vi "CreateABLEDataStructures.vi"(8 "Error In":errorcluster) -> (0 "Error Out":errorcluster, 3 "ABLE Data Structures":T1)   [LabVIEW 2012]
uses:
  ABLEDataStructures.ctl
  HardwareDisplayData.ctl
  BPM.ctl
  ExperimentHardwareData.ctl
  ExperimentData.ctl
  AlarmData.ctl
  AlarmDatum.ctl
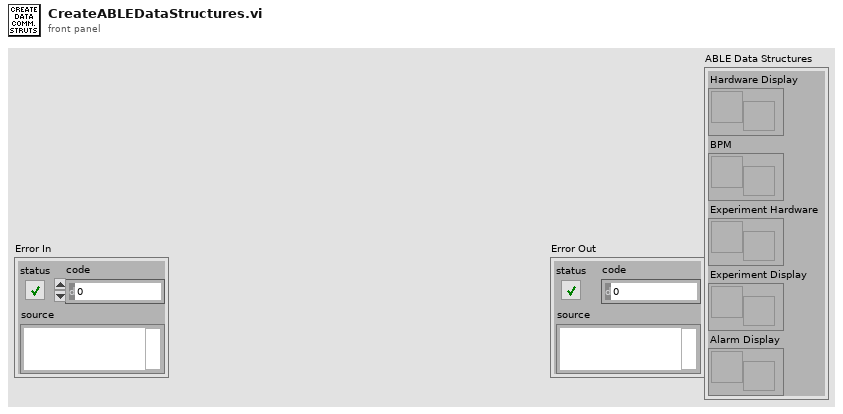
[diagram p1: front panel]
types:
  T1 = typedef "ABLEDataStructures.ctl" = cluster{"Hardware Display":refnum<notifier>, "BPM":refnum<notifier>, "Experiment Hardware":refnum<notifier>, "Experiment Display":refnum<notifier>, "Alarm Display":refnum<notifier>}
  T2 = typedef "AlarmData.ctl" = cluster{"Temperature":T3[]}
  T3 = typedef "AlarmDatum.ctl" = cluster{"Actual":dbl, "Activated?":bool}
  T4 = typedef "ExperimentData.ctl" = cluster{"Flux (ions/s * cm^2)":dbl, "Average Flux (ions/s * cm^2)":dbl, "DPA Rate":dbl, "Average DPA Rate":dbl, "Total Ion Energy (MeV)":dbl, "Total Charge (C)":dbl, "Dose (DPA)":dbl, "Fluence (ions/cm^2)":dbl, "Percent Complete (%)":dbl, "Duration (sec)":dbl}
  T5 = typedef "ExperimentHardwareData.ctl" = cluster{"Beam Current (A)":dbl, "Terminal Voltage (MeV)":dbl}
  T6 = typedef "HardwareDisplayData.ctl" = cluster{"Temperatures (C)":dbl[], "Terminal Voltage (MeV)":dbl, "Currents (A)":dbl[]}
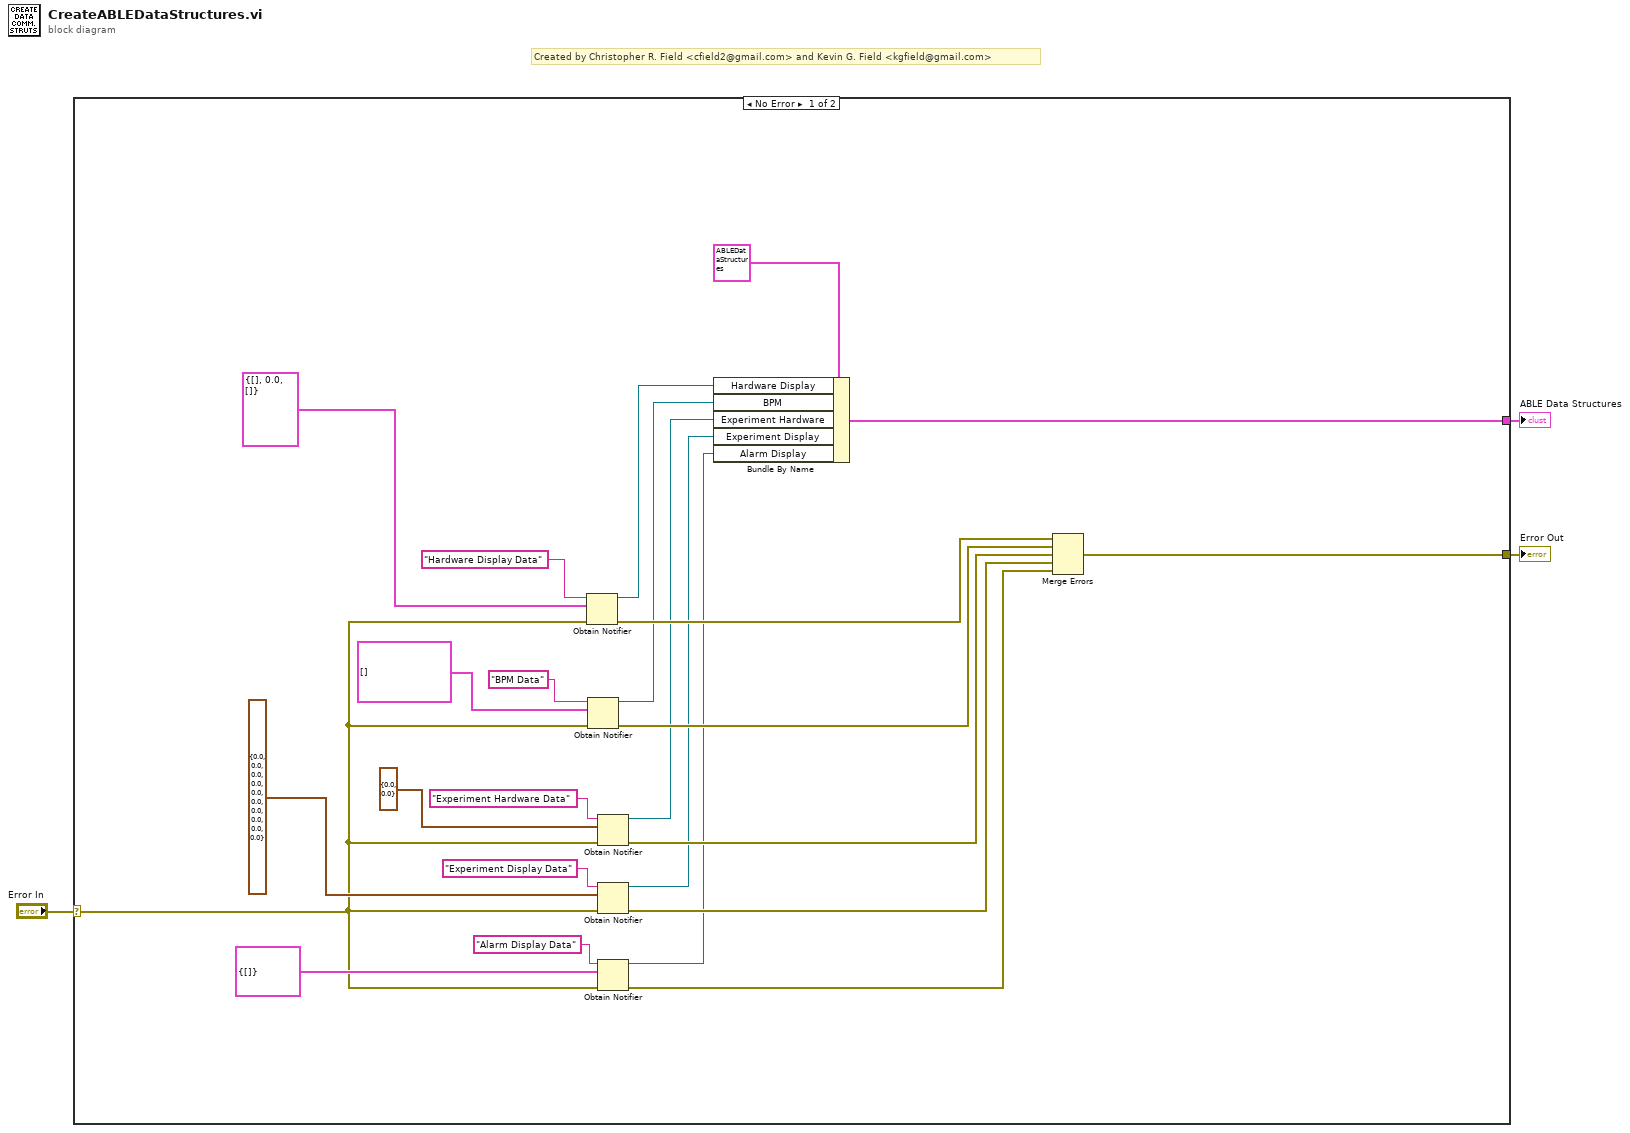
[diagram p0: block diagram]
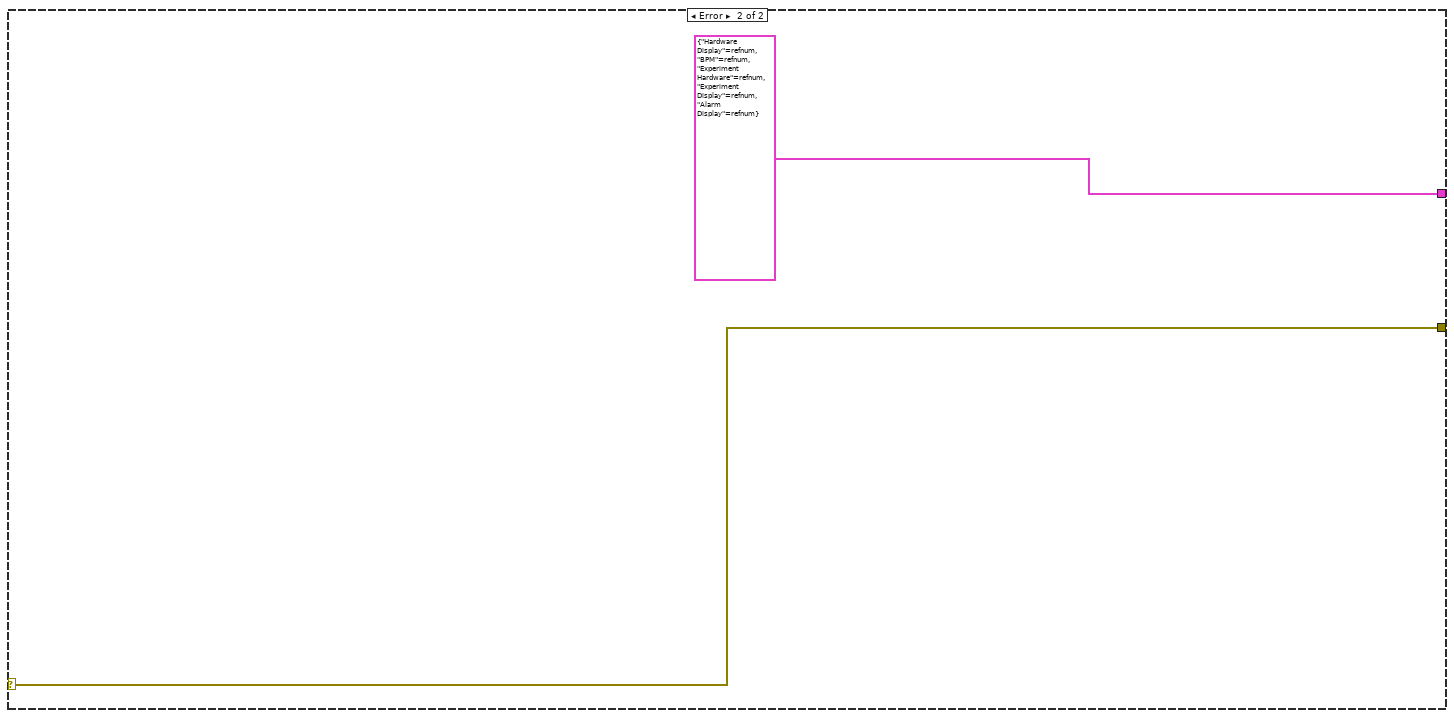
[diagram p2: hidden frame]
diagram:
  # "Created by Christopher R. Field <cfield2@gmail.com> and Kevin G. Field <kgfield@gmail.com>"
  n1 = case shown="No Error" "Error In" {
    selector: "Error In" -> [w6 w29]
    tunnel: [w26 w29] -> w2
    tunnel: [w24 T1 {"Hardware Display"=refnum, "BPM"=refnum, "Experiment Hardware"=refnum, "Experiment Display"=refnum, "Alarm Display"=refnum} ("Data Communication Structures")] -> w1
    frame No Error {
      n2 = Obtain Notifier(name (unnamed)="Hardware Display Data", notification data type=T6 {"Temperatures (C)"=[], "Terminal Voltage (MeV)"=0.0, "Currents (A)"=[]} ("Display Data"), error in (no error)=w6) -> (notifier out=w17:refnum<notifier>, error out=w23:errorcluster)  [unwired: 1 in, 1 out]
      n3 = Obtain Notifier(name (unnamed)="BPM Data", notification data type=cluster{dbl[], "Beam Profile":dbl[]}[] [] ("BPM"), error in (no error)=w6) -> (notifier out=w20:refnum<notifier>, error out=w21:errorcluster)  [unwired: 1 in, 1 out]
      n4 = Obtain Notifier(name (unnamed)="Experiment Hardware Data", notification data type=T5 {"Beam Current (A)"=0.0, "Terminal Voltage (MeV)"=0.0} ("Experiment Hardware Data"), error in (no error)=w6) -> (notifier out=w11:refnum<notifier>, error out=w14:errorcluster)  [unwired: 1 in, 1 out]
      n5 = Obtain Notifier(name (unnamed)="Experiment Display Data", notification data type=T4 {"Flux (ions/s * cm^2)"=0.0, "Average Flux (ions/s * cm^2)"=0.0, "DPA Rate"=0.0, "Average DPA Rate"=0.0, "Total Ion Energy (MeV)"=0.0, "Total Charge (C)"=0.0, "Dose (DPA)"=0.0, "Fluence (ions/cm^2)"=0.0, "Percent Complete (%)"=0.0, "Duration (sec)"=0.0} ("Experiment Data"), error in (no error)=w6) -> (notifier out=w9:refnum<notifier>, error out=w10:errorcluster)  [unwired: 1 in, 1 out]
      n6 = Obtain Notifier(name (unnamed)="Alarm Display Data", notification data type=T2 {"Temperature"=[]} ("Alarm Data"), error in (no error)=w6) -> (notifier out=w4:refnum<notifier>, error out=w5:errorcluster)  [unwired: 1 in, 1 out]
      n7 = Bundle By Name(cluster=T1 {"Hardware Display"=refnum, "BPM"=refnum, "Experiment Hardware"=refnum, "Experiment Display"=refnum, "Alarm Display"=refnum} ("Data Communication Structures"), "Hardware Display"=w17, "BPM"=w20, "Experiment Hardware"=w11, "Experiment Display"=w9, "Alarm Display"=w4) -> (w24:T1)
      n8 = Merge Errors(w23, w21, w14, w10, w5) -> (w26:errorcluster)
    }
    frame Error {
    }
  }
  "Error Out" <- w2
  "ABLE Data Structures" <- w1
